vi "nPoints Concept - Digital Temp.vi"() -> ()   [LabVIEW 2014]
panel:
  out "T_C":dbl(slide) scale=0.0..100.0
  out "T_B":dbl(slide) scale=0.0..100.0
  in  "Stop Button":bool
  out "T_A":dbl(slide) scale=0.0..100.0
  in  "Response Hold":dbl=1.0
  in  "Response time":dbl=2.0
  out "temp":dbl=23.7
  in  "Command Hold":dbl=1.0
  in  "Temp_C":bool
  in  "Temp_B":bool
  in  "Temp_A":bool
  in  "Messege timing":dbl=2.0
  out "SCL N3":u32(colorbox)
  out "SCL N2":u32(colorbox)
  out "SCL N1":u32(colorbox)
  in  "Master":bool
  in  "Message":enum16{"Config", "Tset", "Thyst", "Temp?"}(ring)
  in  "Send":bool
  in  "Device Select":enum16{"Temp_A", "Temp_B", "Temp_C"}(ring)
  out "SCL (Clock)":u32(colorbox)
  out "SCL S3":u32(colorbox)
  out "SCL S2":u32(colorbox)
  out "SCL S1":u32(colorbox)
  out "SDA S3":dbl(slide) scale=0.0..10.0
  out "SDA S2":dbl(slide) scale=0.0..10.0
  out "SDA S1":dbl(slide) scale=0.0..10.0
  out "SDA (Data)":dbl(slide) scale=0.0..50.0
  # "Digital Temperture Sensor"
  # "Temp B"
  # "Temp C"
  # "Temp A"
  # "VDD (3.3V)"
  # "GND"
  # "Rp"
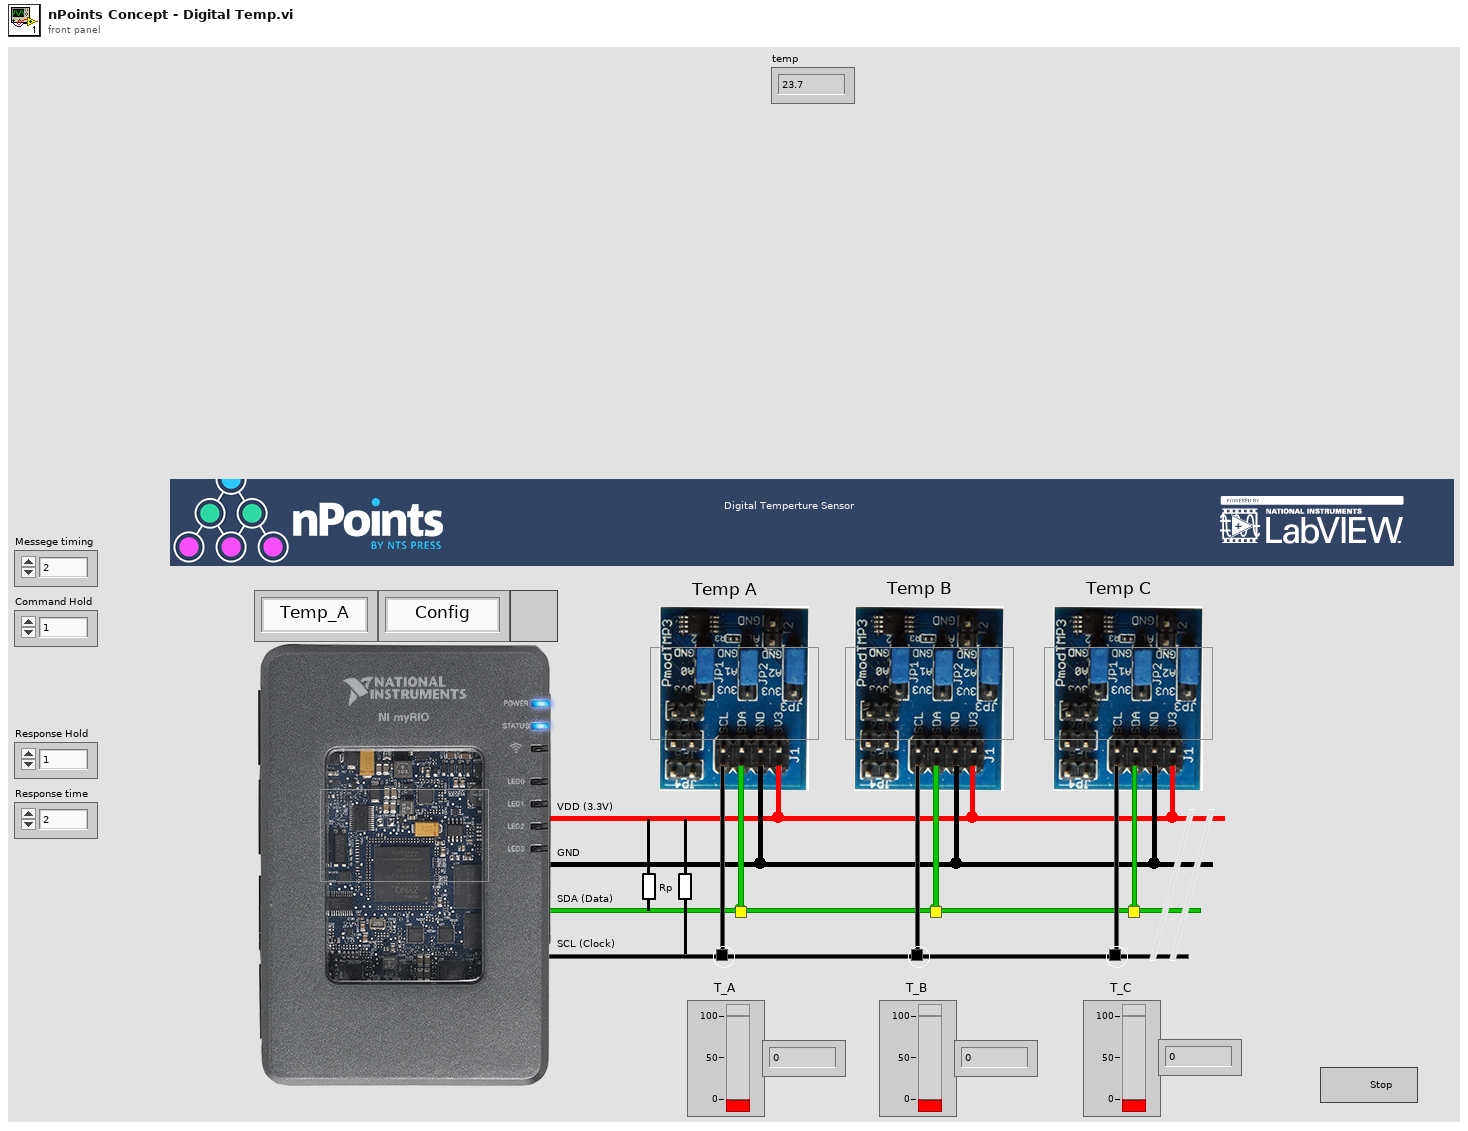
[diagram p1: front panel]
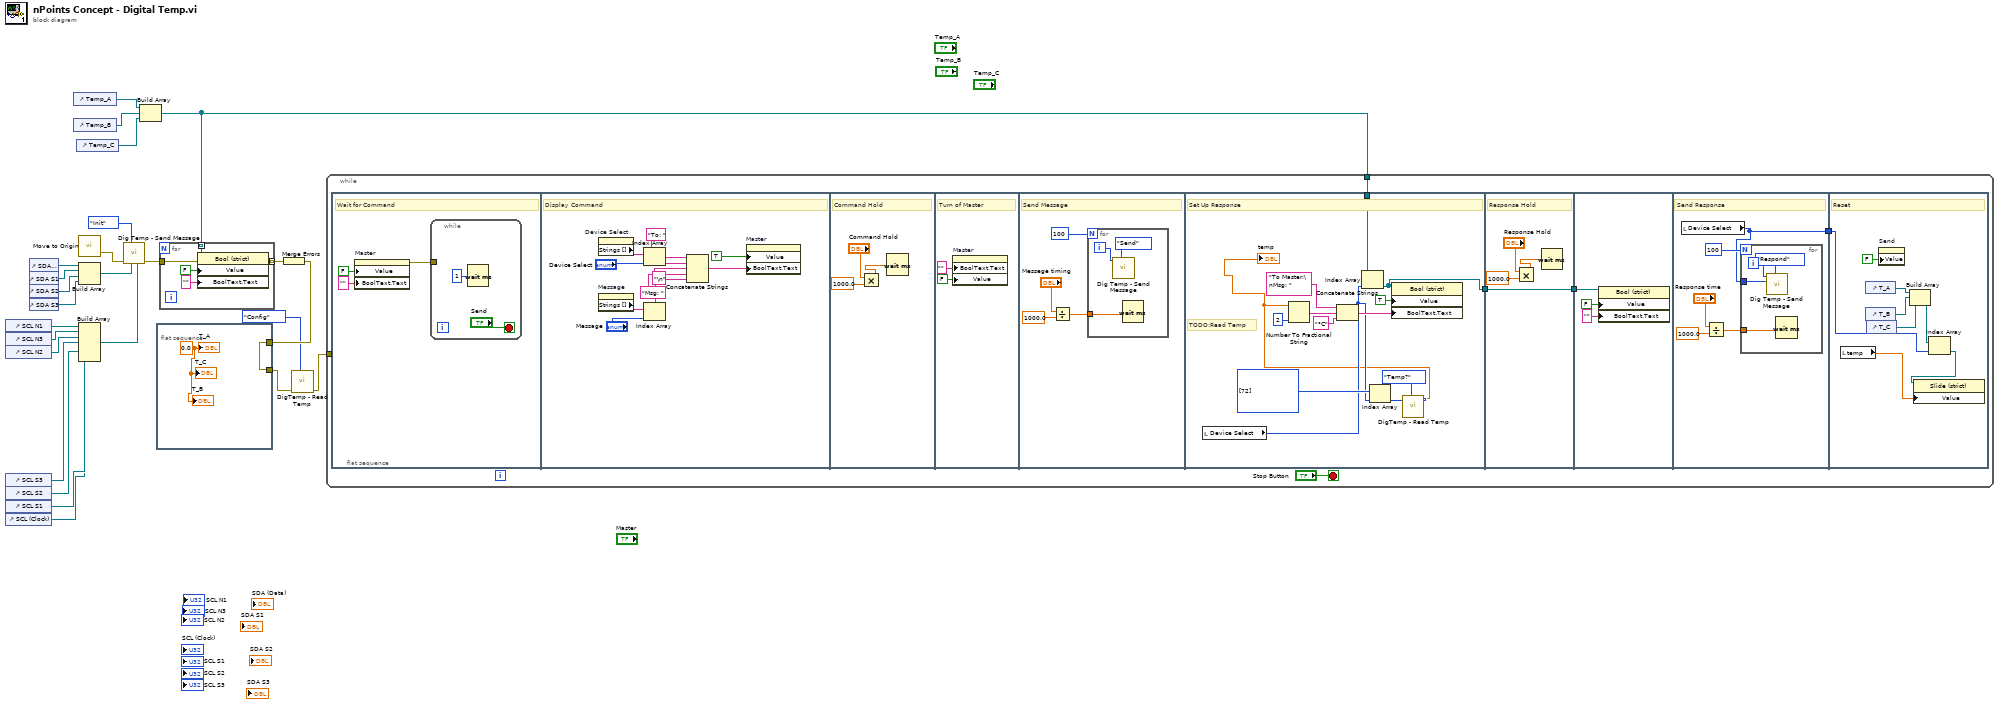
[diagram p0: block diagram]
diagram:
  n1 = control-ref of="SCL N1"() -> (w25:refnum<vi>)
  n2 = control-ref of="SCL N3"() -> (w24:refnum<vi>)
  n3 = control-ref of="SCL N2"() -> (w23:refnum<vi>)
  n4 = control-ref of="SCL S3"() -> (w22:refnum<vi>)
  n5 = control-ref of="SCL S2"() -> (w21:refnum<vi>)
  n6 = control-ref of="SCL S1"() -> (w20:refnum<vi>)
  n7 = control-ref of="SCL (Clock)"() -> (w19:refnum<vi>)
  n8 = control-ref of="SDA (Data)"() -> (w15:refnum<vi>)
  n9 = control-ref of="SDA S1"() -> (w16:refnum<vi>)
  n10 = control-ref of="SDA S2"() -> (w17:refnum<vi>)
  n11 = control-ref of="SDA S3"() -> (w18:refnum<vi>)
  n12 = control-ref of="Temp_A"() -> (w10:refnum<vi>)
  n13 = control-ref of="Temp_B"() -> (w6:refnum<vi>)
  n14 = control-ref of="Temp_C"() -> (w5:refnum<vi>)
  n15 = call <userlib>:"Move to Origin.vi"() -> ("Error Out"=w11:errorcluster)  [unwired: 3 in]
  n16 = Build Array(w15, w16, w17, w18) -> (w13:refnum<vi>[])
  n17 = Build Array(w25, w24, w23, w22, w21, w20, w19) -> (w12:refnum<vi>[])
  n18 = call "Dig Temp - Send Message.vi"("Clock Wire Refs"=w12, "SDA Refs"=w13, "State"=enum16{"Init", "Send", "Respond"}."Init", "error in (no error)"=w11) -> ("error out"=w8:errorcluster)  [unwired: 7 in]
  n19 = Build Array(w10, w6, w5) -> (w9:refnum<vi>[])
  n20 = flat-sequence {
    tunnel: w4 -> [w26]
    tunnel: [w26] -> w3
    frame #0 {
      w27 = 0.0 ("T1")
      "T_B" <- w27
      "T_C" <- w27
      "T_A" <- w27
    }
  }
  n21 = for {
    tunnel: w9 -> [w32] mode=indexing
    tunnel: w8 -> [w29]
    tunnel: [w28] -> w7 mode=indexing
    n22 = property on="Property Node" class="Bool (strict)"(reference=w32, error in=w29, "Value"=FALSE, "BoolText.Text"="" ("Boolean Text.Text")) -> (error out=w28:errorcluster)  [unwired: 1 out]
  }
  n23 = Merge Errors(w7) -> (w4:errorcluster)
  n24 = call "DigTemp - Read Temp.vi"("Mode"=enum16{"Config", "Temp?"}."Config", "error in (no error)"=w3) -> ("error out"=w2:errorcluster)  [unwired: 7 in, 2 out]
  n25 = while {
    tunnel: w9 -> [w37]
    tunnel: w2 -> [_]
    stop <- "Stop Button" stop-if-true
    n26 = flat-sequence {
      tunnel: w37 -> [w72]
      tunnel: [w69] -> w36
      tunnel: w36 -> [w79]
      tunnel: [w79] -> w35
      tunnel: w35 -> [w85]
      tunnel: [w86] -> w33
      tunnel: w33 -> [w97]
      frame #0 {
        # "Wait for Command"
        n27 = property on="Master" class="Bool (strict)"("Value"=FALSE ("Master"), "BoolText.Text"="" ("Boolean Text.Text")) -> (error out=w38:errorcluster)  [unwired: 2 in, 1 out]
        n28 = while {
          tunnel: w38 -> [_]
          stop <- "Send" stop-if-true
          n29 = Wait (ms)(milliseconds to wait=u32 1) -> ()  [unwired: 1 out]
        }
      }
      frame #1 {
        # "Display Command"
        n30 = property on="Device Select" class="Enum (strict)"() -> ("Strings []"=w50:string[])  [unwired: 2 in, 2 out]
        n31 = property on="Message" class="Enum (strict)"() -> ("Strings []"=w51:string[])  [unwired: 2 in, 2 out]
        n32 = Index Array(array=w50, index="Device Select") -> (element=w47:string)
        n33 = Index Array(array=w51, index="Message") -> (element=w44:string)
        n34 = Concatenate Strings("To: " ("Boolean Text.Text"), w47, "\n" ("string"), "Msg: " ("Boolean Text.Text"), w44) -> (w49:string)
        n35 = property on="Master" class="Bool (strict)"("Value"=TRUE ("Master"), "BoolText.Text"=w49) -> ()  [unwired: 2 in, 2 out]
      }
      frame #2 {
        # "Command Hold"
        n36 = Multiply(x="Command Hold", y=1000.0) -> (x*y=w54:dbl)
        n37 = Wait (ms)(milliseconds to wait=w54) -> ()  [unwired: 1 out]
      }
      frame #3 {
        # "Turn of Master"
        n38 = property on="Master" class="Bool (strict)"("BoolText.Text"="" ("Boolean Text.Text"), "Value"=FALSE ("Master")) -> ()  [unwired: 2 in, 2 out]
      }
      frame #4 {
        # "Send Message"
        n39 = Divide(x="Messege timing", y=1000.0) -> (x/y=w59:dbl)
        n40 = for {
          N: 100 -> [_]
          tunnel: w59 -> [w65]
          i -> [w64]
          n41 = call "Dig Temp - Send Message.vi"("State"=enum16{"Init", "Send", "Respond"}."Send", "t (0-100)"=w64) -> ()  [unwired: 9 in, 1 out]
          n42 = Wait (ms)(milliseconds to wait=w65) -> ()  [unwired: 1 out]
        }
      }
      frame #5 {
        # "TODO:Read Temp"
        # "Set Up Response"
        n43 = local read "Device Select"() -> (w70:enum16{"Temp_A", "Temp_B", "Temp_C"})
        n44 = Index Array(array=w72, index=w70) -> (element=w69:refnum<vi>)
        n45 = Index Array(array=u8[] [72], index=w70) -> (element=w68:u8)
        n46 = call "DigTemp - Read Temp.vi"("Mode"=enum16{"Config", "Temp?"}."Temp?", "PmodTMP3 address (x48)"=w68) -> ("Temp"=w67:dbl)  [unwired: 7 in, 2 out]
        "temp" <- w67
        n47 = Number To Fractional String(number=w67, precision (6)=i16 2) -> (F-format string=w76:string)  [unwired: 2 in]
        n48 = Concatenate Strings("To Master:\nMsg: " ("Boolean Text.Text"), w76, "°C" ("Boolean Text.Text")) -> (w78:string)
        n49 = property on="Property Node" class="Bool (strict)"(reference=w69, "Value"=TRUE ("Master"), "BoolText.Text"=w78) -> ()  [unwired: 1 in, 2 out]
      }
      frame #6 {
        # "Response Hold"
        n50 = Multiply(x="Response Hold", y=1000.0) -> (x*y=w82:dbl)
        n51 = Wait (ms)(milliseconds to wait=w82) -> ()  [unwired: 1 out]
      }
      frame #7 {
        n52 = property on="Property Node" class="Bool (strict)"(reference=w85, "Value"=FALSE, "BoolText.Text"="" ("Boolean Text.Text")) -> ()  [unwired: 1 in, 2 out]
      }
      frame #8 {
        # "Send Response"
        n53 = local read "Device Select"() -> (w86:enum16{"Temp_A", "Temp_B", "Temp_C"})
        n54 = Divide(x="Response time", y=1000.0) -> (x/y=w90:dbl)
        n55 = for {
          N: 100 -> [_]
          tunnel: w90 -> [w94]
          tunnel: w86 -> [w91]
          i -> [w93]
          n56 = call "Dig Temp - Send Message.vi"("State"=enum16{"Init", "Send", "Respond"}."Respond", "Device Select"=w91, "t (0-100)"=w93) -> ()  [unwired: 8 in, 1 out]
          n57 = Wait (ms)(milliseconds to wait=w94) -> ()  [unwired: 1 out]
        }
      }
      frame #9 {
        # "Reset"
        n58 = local read "temp"() -> (w98:dbl)
        n59 = control-ref of="T_A"() -> (w101:refnum<vi>)
        n60 = control-ref of="T_B"() -> (w96:refnum<vi>)
        n61 = control-ref of="T_C"() -> (w95:refnum<vi>)
        n62 = property on="Send" class="Bool (strict)"("Value"=FALSE ("Send")) -> ()  [unwired: 2 in, 2 out]
        n63 = Build Array(w101, w96, w95) -> (w100:refnum<vi>[])
        n64 = Index Array(array=w100, index=w97) -> (element=w99:refnum<vi>)
        n65 = property on="Property Node" class="Slide (strict)"(reference=w99, "Value"=w98) -> ()  [unwired: 1 in, 2 out]
      }
    }
  }
